vi "Add New Report Event.vi"(8 "error in":errorcluster, 11 "Report Generator in":refnum<class "Report Generator.lvclass">) -> (0 "error out":errorcluster, 3 "Report Generator out":refnum<class "Report Generator.lvclass">)   [LabVIEW 2019, in "Report Generator.lvlib" / "Report Generator.lvclass"]
uses:
  Library/Report Generator.lvclass
  C:/Users/Public/Documents/Development/builds/Engine/Engine.lvlibp/Project/Engine.lvclass
  builds/Engine/Engine.lvlibp/Accessors/Read Report Queue.vi
  builds/Tools/QDMH.lvlibp/QDMH.lvclass
  builds/Engine/Engine.lvlibp/Project/Engine.lvclass
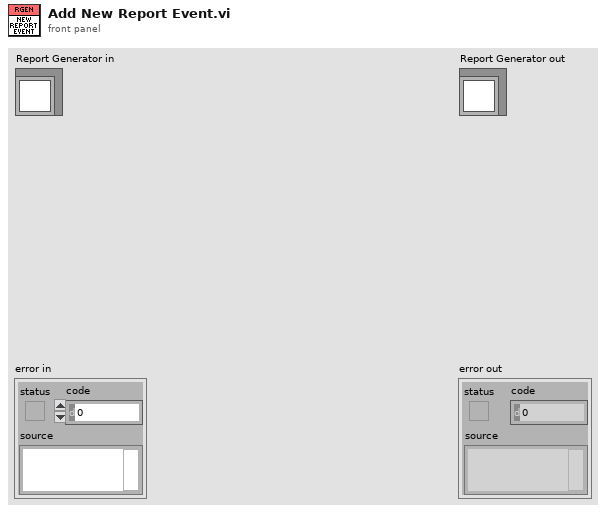
[diagram p1: front panel]
types:
  T1 = cluster{"seconds since 1Jan1904":timestamp, string, string, string}
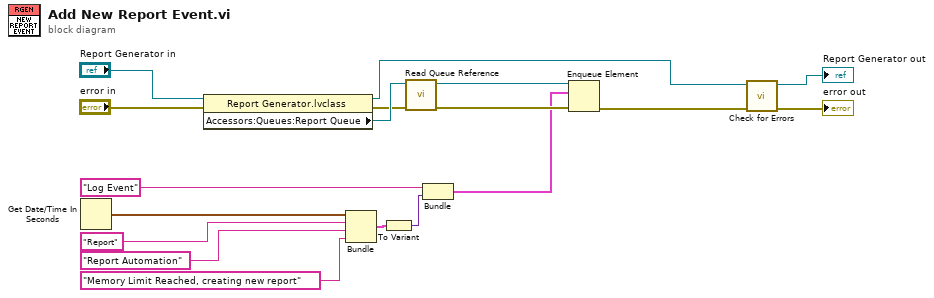
[diagram p0: block diagram]
diagram:
  n1 = Get Date/Time In Seconds() -> (seconds since 1Jan1904=w9:timestamp)
  n2 = property class="Report Generator.lvclass"(reference="Report Generator in", error in="error in") -> (reference out=w11:refnum<class "Report Generator.lvclass">, error out=w17:errorcluster, "Accessors:Queues:Report Queue"=w18:refnum<class "QDMH.lvclass">)
  n3 = Bundle("seconds since 1Jan1904"=w9, "Report", "Report Automation", "Memory Limit Reached, creating new report") -> (w5:T1)  [unwired: 1 in]
  n4 = To Variant(anything=w5) -> (Variant=w4:variant)
  n5 = call "Read Queue Reference.vi"("error in"=w17, "QDMH in"=w18) -> ("error out"=w13:errorcluster, "Queue Reference"=w12:refnum<queue>)  [unwired: 7 in, 1 out]
  n6 = Bundle("Log Event", "Variant"=w4) -> (w1:cluster{string, "Variant":variant})  [unwired: 1 in]
  n7 = Enqueue Element(queue=w12, element=w1, error in (no error)=w13) -> (error out=w10:errorcluster)  [unwired: 1 in, 2 out]
  n8 = call "Check for Errors.vi"("error in"=w10, "Engine in"=w11) -> ("error out"=→"error out":errorcluster, "Engine out"=→"Report Generator out":refnum<class "Report Generator.lvclass">)  [unwired: 8 in]
